vi "Baidu_Voice.vi"() -> ()   [LabVIEW 2013]
uses:
  <vilib>/httpClient/POSTBuffer.vi
  <vilib>/httpClient/LabVIEWHTTPClient.lvlib
panel:
  out "decimal integer string":string
  out "string out (base64-encoded)":string
  out "body":string
  out "headers":string
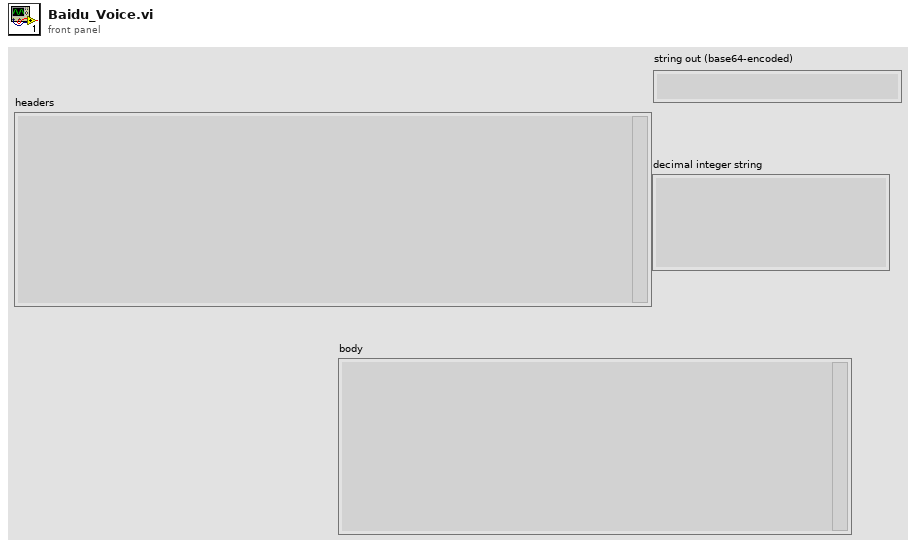
[diagram p1: front panel]
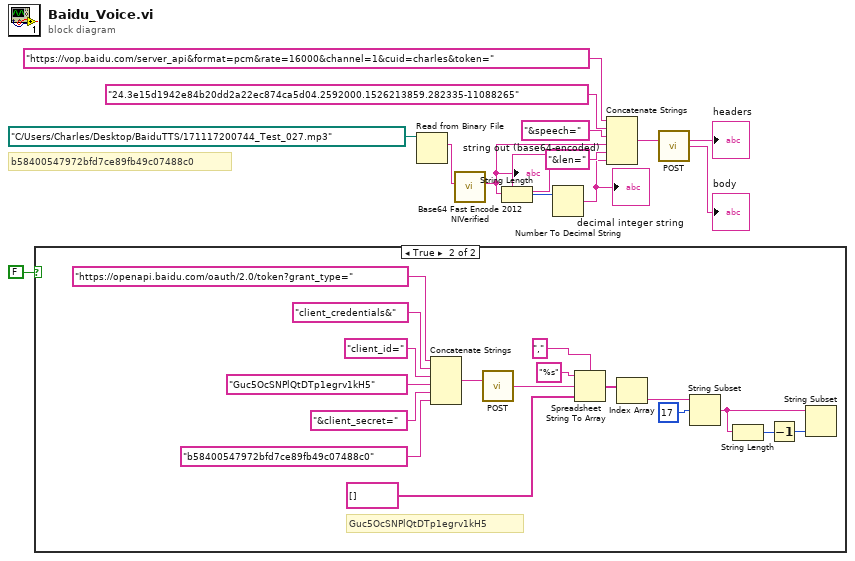
[diagram p0: block diagram]
diagram:
  # "b58400547972bfd7ce89fb49c07488c0"
  n1 = case shown="True" FALSE {
    frame False {
    }
    frame True {
      # "Guc5OcSNPlQtDTp1egrv1kH5"
      n2 = Concatenate Strings("https://openapi.baidu.com/oauth/2.0/token?grant_type=" ("string"), "client_credentials&" ("string"), "client_id=" ("string"), "Guc5OcSNPlQtDTp1egrv1kH5" ("string"), "&client_secret=" ("string"), "b58400547972bfd7ce89fb49c07488c0" ("string")) -> (w30:string)
      n3 = call-poly <vilib>:"POST.vi"("url"=w30) -> ("body"=w14:string)  [unwired: 11 in, 3 out]
      n4 = Spreadsheet String To Array(delimiter (Tab)=",", format string="%s", spreadsheet string=w14, array type (2D Dbl)=string[] []) -> (array=w20:string[])
      n5 = Index Array(array=w20) -> (element=w19:string)  [unwired: 1 in]
      n6 = String Subset(string=w19, offset (0)=17) -> (substring=w17:string)  [unwired: 1 in]
      n7 = String Length(string=w17) -> (length=w16:i32)
      n8 = Decrement(x=w16) -> (x-1=w15:i32)
      n9 = String Subset(string=w17, length (rest)=w15) -> ()  [unwired: 1 in, 1 out]
    }
  }
  n10 = Read from Binary File(11:path "C:/Users/Charles/Desktop/BaiduTTS/171117200744_Test_027.mp3" ("file")) -> (2:w2:string)  [unwired: 5 in, 3 out]
  n11 = call "Base64 Fast Encode 2012 NIVerified.vi"("string in (not encoded)"=w2) -> ("string out (base64-encoded)"=w1:string)  [unwired: 9 in, 1 out]
  "string out (base64-encoded)" <- w1
  n12 = String Length(string=w1) -> (length=w4:i32)
  n13 = Number To Decimal String(number=w4) -> (decimal integer string=w3:string)  [unwired: 1 in]
  "decimal integer string" <- w3
  n14 = Concatenate Strings("https://vop.baidu.com/server_api&format=pcm&rate=16000&channel=1&cuid=charles&token=" ("url"), "24.3e15d1942e84b20dd2a22ec874ca5d04.2592000.1526213859.282335-11088265" ("Access_Token"), "&speech=" ("string"), w1, "&len=" ("string"), w3) -> (w12:string)
  n15 = call-poly <vilib>:"POST.vi"("url"=w12) -> ("headers"=→"headers":string, "body"=→"body":string)  [unwired: 11 in, 2 out]
